vi "Initialize.vi"(8 "error in (no error)":errorcluster, 11 "Test Step Controller":refnum<class "Server Controller.lvclass">) -> (0 "error out":errorcluster, 3 "Test Step Controller Out":refnum<class "Server Controller.lvclass">)   [LabVIEW 2016, in "Server Controller.lvlib" / "Server Controller.lvclass"]
uses:
  Server Controller.lvclass
  \\Mac\Home/Documents/MAL-Framework/user.lib/Common Components/Controller/Controller.lvclass
  C:/Program Files (x86)/National Instruments/LabVIEW 2016/vi.lib/ActorFramework/Actor/Actor.lvclass
  MAL-Framework/user.lib/Common Components/Controller/Controller.lvclass/Controller.ctl
  <vilib>/ActorFramework/Actor/Actor.lvclass/Actor.ctl
  <vilib>/ActorFramework/Message Enqueuer/Message Enqueuer.lvclass/Message Enqueuer.ctl
  <vilib>/ActorFramework/Message Enqueuer/Init from Existing Queue.vi
  <vilib>/ActorFramework/Message Enqueuer/Enqueue.vi
  <vilib>/ActorFramework/Stop Msg/Stop Msg.lvclass
  C:/Program Files (x86)/National Instruments/LabVIEW 2016/vi.lib/ActorFramework/Message/Message.lvclass
  <vilib>/ActorFramework/Message Priority Queue/Priority Enqueue.vi
  <vilib>/ActorFramework/Message Enqueuer/Message Enqueuer.lvclass
  <vilib>/ActorFramework/Actor/Actor.lvclass
  MAL-Framework/user.lib/Common Components/Controller/Controller.lvclass
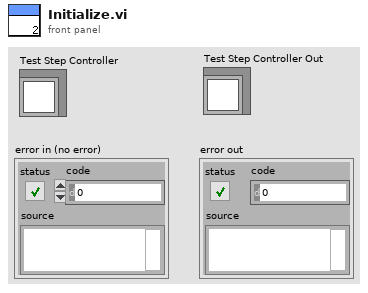
[diagram p1: front panel]
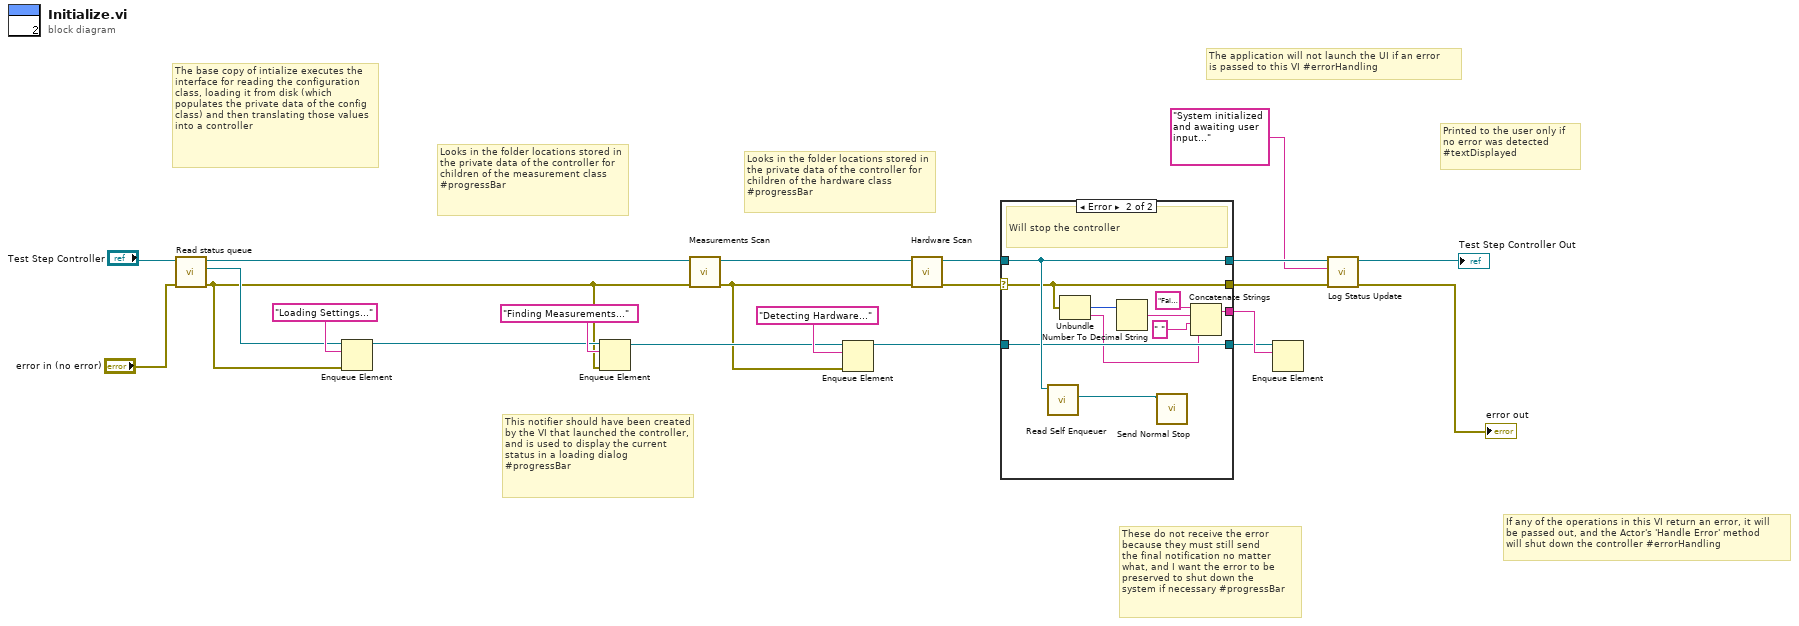
[diagram p0: block diagram]
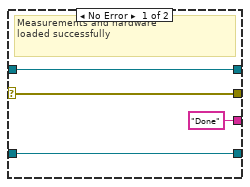
[diagram p2: hidden frame]
diagram:
  # "The base copy of intialize executes the interface for reading the configuration class, loading it from disk (which populates the private data of the config class) and then translating those values into a controller"
  # "Printed to the user only if \nno error was detected\n#textDisplayed"
  # "This notifier should have been created by the VI that launched the controller, and is used to display the current status in a loading dialog #progressBar"
  # "Looks in the folder locations stored in the private data of the controller for children of the hardware class \n#progressBar"
  # "Looks in the folder locations stored in the private data of the controller for children of the measurement class #progressBar"
  # "These do not receive the error\nbecause they must still send \nthe final notification no matter \nwhat, and I want the error to be \npreserved to shut down the \nsystem if necessary #progressBar"
  # "The application will not launch the UI if an error\nis passed to this VI #errorHandling"
  # "If any of the operations in this VI return an error, it will\nbe passed out, and the Actor's 'Handle Error' method \nwill shut down the controller #errorHandling"
  n1 = call "Read status queue.vi"("error in (no error)"="error in (no error)", "Controller in"="Test Step Controller") -> ("error out"=w1:errorcluster, "status queue"=w3:refnum<queue>, "Controller out"=w2:refnum<class "Server Controller.lvclass">)  [unwired: 7 in]
  n2 = Enqueue Element(queue=w3, element="Loading Settings..." ("notification"), error in (no error)=w1) -> (queue out=w13:refnum<queue>)  [unwired: 1 in, 2 out]
  n3 = Enqueue Element(queue=w13, element="Finding Measurements..." ("notification"), error in (no error)=w1) -> (queue out=w16:refnum<queue>)  [unwired: 1 in, 2 out]
  n4 = call-dynamic "Measurements Scan.vi"("error in (no error)"=w1, "Controller in"=w2) -> ("error out"=w11:errorcluster, "Controller out"=w15:refnum<class "Server Controller.lvclass">)  [unwired: 8 in]
  n5 = Enqueue Element(queue=w16, element="Detecting Hardware..." ("notification"), error in (no error)=w11) -> (queue out=w18:refnum<queue>)  [unwired: 1 in, 2 out]
  n6 = call-dynamic "Hardware Scan.vi"("error in (no error)"=w11, "Controller in"=w15) -> ("error out"=w22:errorcluster, "Controller out"=w19:refnum<class "Server Controller.lvclass">)  [unwired: 8 in]
  n7 = case shown="Error" w22 {
    selector: w22 -> [w24 w31]
    tunnel: w18 -> [w23 w35]
    tunnel: [w24 w31] -> w7
    tunnel: [w26 w36] -> w10
    tunnel: w19 -> [w26 w36]
    tunnel: ["Done" ("notification") w32] -> w21
    tunnel: [w23 w35] -> w20
    frame No Error {
      # "Measurements and hardware\nloaded successfully"
    }
    frame Error {
      # "Will stop the controller"
      n8 = call <vilib>:"Read Self Enqueuer.vi"("Actor"=w36) -> ("Self Enqueuer"=w34:refnum<class "Message Enqueuer.lvclass">)  [unwired: 10 in]
      n9 = Unbundle(w31) -> ("code"=w29:i32, "source"=w27:string)  [unwired: 1 out]
      n10 = Number To Decimal String(number=w29) -> (decimal integer string=w30:string)  [unwired: 1 in]
      n11 = call <vilib>:"Send Normal Stop.vi"("Message Enqueuer"=w34) -> ()  [unwired: 10 in, 1 out]
      n12 = Concatenate Strings("Failure. Cancelling Launch. Error: " ("notification"), w30, " " ("string"), w27) -> (w32:string)
    }
  }
  n13 = Enqueue Element(queue=w20, element=w21) -> ()  [unwired: 2 in, 3 out]
  n14 = call-dynamic "Log Status Update.vi"("error in (no error)"=w7, "String"="System initialized and awaiting user input...", "Controller in"=w10) -> ("error out"=→"error out":errorcluster, "Controller out"=→"Test Step Controller Out":refnum<class "Server Controller.lvclass">)  [unwired: 7 in]
